vi "VisionBallTracking.vi"(10 "Refnum in":T1, 11 "Refnum in":T2) -> (2 "Position":cluster{"X":sgl, "Y":sgl}, 3 "Refnum out":T1)   [LabVIEW 2021]
uses:
  <vilib>/vision/Image Controls.llb/IMAQ Image.ctl
  <vilib>/userDefined/High Color/IMAQdx.ctl
  <vilib>/vision/driver/IMAQdx.llb/IMAQdx Buffer Number Mode.ctl
  <vilib>/vision/Management.llb/Cast Image 2 Method.ctl
  <vilib>/vision/Shape Detection.llb/ShapeDetectionMatchOptions.ctl
  <vilib>/vision/Pattern Matching.llb/IMAQ Match Range Setting.ctl
  <vilib>/vision/driver/NI_Vision_Acquisition_Software.lvlib
  <vilib>/vision/NI_Vision_Development_Module.lvlib
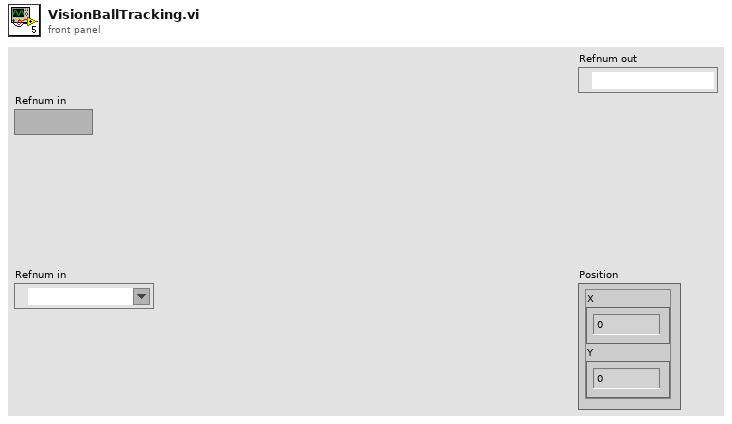
[diagram p1: front panel]
types:
  T1 = typedef "IMAQdx.ctl" = refnum<k21>
  T2 = typedef "IMAQ Image.ctl" = refnum<image>
  T3 = typedef "ShapeDetectionMatchOptions.ctl" = cluster{"Rotation":bool, "Scale":bool, "Occlusion":bool, "Range Settings":T4[]}
  T4 = typedef "IMAQ Match Range Setting.ctl" = cluster{"Match Constraints":u32, "Min":dbl, "Max":dbl}
  T5 = typedef "IMAQ Rectangle" = cluster{"Left":i32, "Top":i32, "Right":i32, "Bottom":i32, "Rotation":dbl}
  T6 = typedef "Cast Image 2 Method.ctl" = u32
  T7 = typedef "Image Type" = u32
  T8 = typedef "NI_Vision_Acquisition_Software.lvlib/IMAQdx Buffer Number Mode.ctl" = enum32{"Next", "Last", "Buffer Number", "Every", "Last New"}
  T9 = typedef "ROI Descriptor" = cluster{"Global Rectangle":i32[], "Contours":cluster{"ID":enum32{"External", "Internal"}, "Type":u32, "Coordinates":i32[]}[]}
  T10 = cluster{"Position":cluster{"X":sgl, "Y":sgl}, "Radius":dbl, "Score":dbl}[]
  T11 = cluster{"Position":cluster{"X":sgl, "Y":sgl}, "Radius":dbl, "Score":dbl}
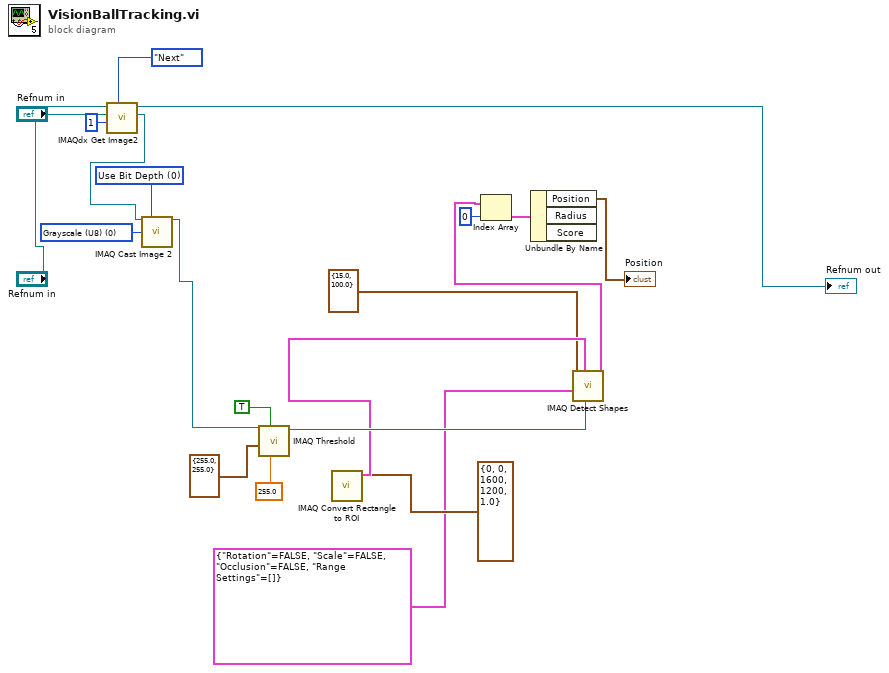
[diagram p0: block diagram]
diagram:
  w7 = T6 0 items=["Use Bit Depth", "Shift", "Use Lookup Table"] ("Method")
  w6 = T7 0 items=["Grayscale (U8)", "Grayscale (I16)", "Grayscale (SGL)", "Complex (CSG)", "RGB (U32)", "HSL (U32)", "RGB (U64)", "Grayscale (U16)"] ("Image Type")
  n1 = call <vilib>:"IMAQdx Get Image2.vi"("Buffer Number Mode (Next)"=IMAQdx_Buffer_Number_Mode."Next", "Buffer Number In"=u32 1, "Image In"="Refnum in", "Session In"="Refnum in") -> ("Image Out"=w20:T2, "Session Out"=→"Refnum out":T1)  [unwired: 4 in, 2 out]
  n2 = call "IMAQ Cast Image 2"("Image Src"=w20, "Method"=w7, "Image Type"=w6) -> ("Image Dst Out"=w8:T2)  [unwired: 11 in, 1 out]
  n3 = call "IMAQ Threshold"("Replace Value"=sgl 255.0, "Keep/Replace Value (Replace)"=TRUE, "Range"=cluster{"Upper value":sgl, "Lower value":sgl} {"Upper value"=255.0, "Lower value"=255.0}, "Image Src"=w8) -> ("Image Dst Out"=w12:T2)  [unwired: 6 in, 1 out]
  n4 = call "IMAQ Convert Rectangle to ROI"("Rectangle"=T5 {"Left"=0, "Top"=0, "Right"=1600, "Bottom"=1200, "Rotation"=1.0}) -> ("ROI Descriptor"=w11:T9)  [unwired: 8 in, 1 out]
  n5 = call-poly "IMAQ Detect Shapes"("ROI Descriptor"=w11, "Match Options"=T3 {"Rotation"=FALSE, "Scale"=FALSE, "Occlusion"=FALSE, "Range Settings"=[]}, "Circle Descriptor"=cluster{"Min Radius":dbl, "Max Radius":dbl} {"Min Radius"=15.0, "Max Radius"=100.0}, "Image"=w12) -> ("Circles"=w17:T10)  [unwired: 5 in, 2 out]
  n6 = Index Array(array=w17, index=0) -> (element=w19:T11)
  n7 = Unbundle By Name(w19) -> ("Position"=→"Position":cluster{"X":sgl, "Y":sgl})  [unwired: 2 out]
